vi "Client UI.vi"(8 "error in (no error)":errorcluster, 11 "Chat Client in":refnum<class "Chat Client.lvclass">) -> (0 "error out":errorcluster, 3 "Chat Client out":refnum<class "Chat Client.lvclass">)   [LabVIEW 2020, in "Chat Client.lvclass"]
uses:
  Chat Client.lvclass
  Chat Client.lvclass/Chat Client.ctl
  Stream-TCP/TCP Client/TCP Client.lvclass
panel:
  in  "Send":bool
  in  "Message":string
  out "Log":string
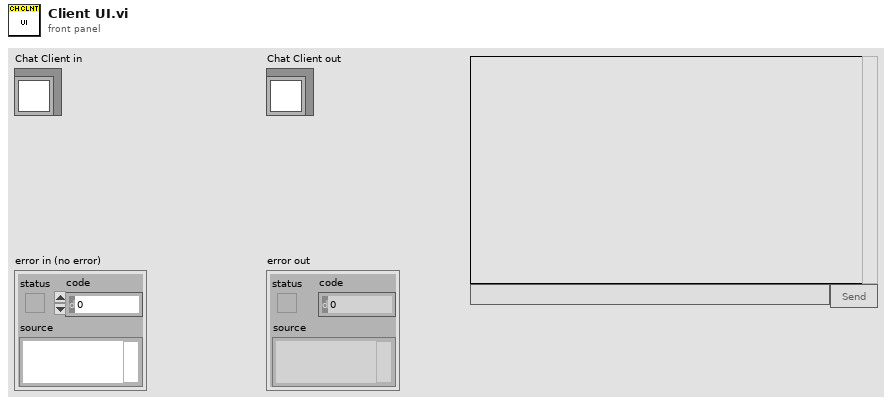
[diagram p1: front panel]
types:
  T1 = enum8{"Enabled", "Disabled", "Disabled and Grayed Out"}
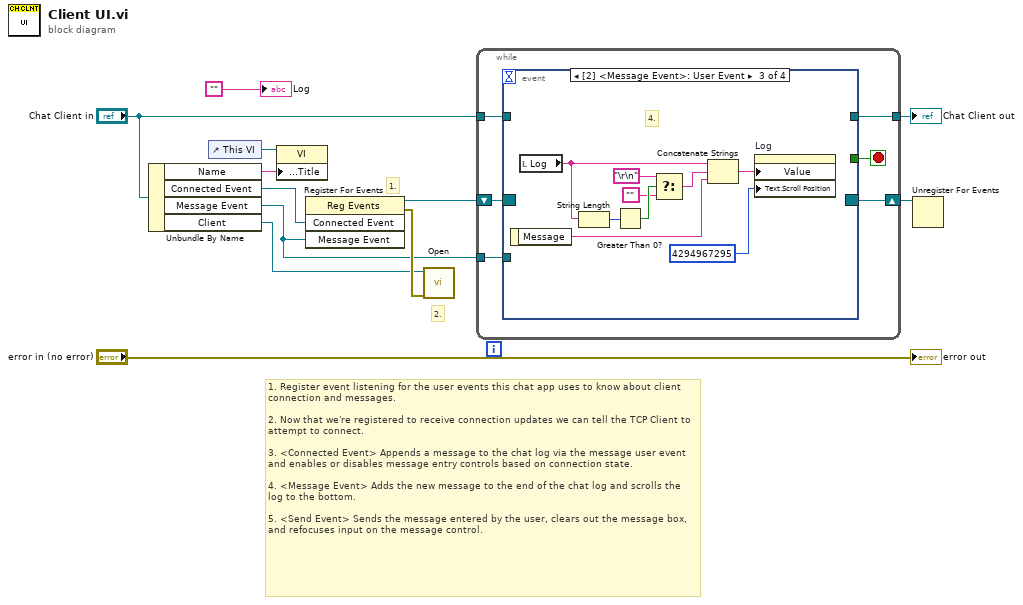
[diagram p0: block diagram]
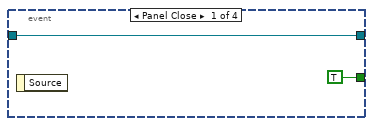
[diagram p2: hidden frame]
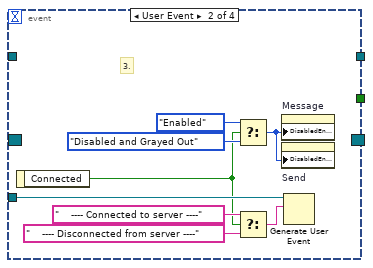
[diagram p3: hidden frame]
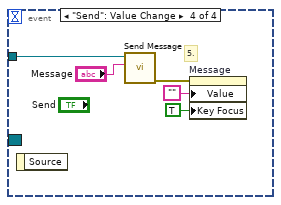
[diagram p4: hidden frame]
diagram:
  # "1. Register event listening for the user events this chat app uses to know about client connection and messages.\n\n2. Now that we're registered to receive connection updates we can tell the TCP Client to attempt to connect.\n\n3. <Connected Event> Appends a message to the chat log via the message user event and enables or disables message entry controls based on connection state.\n\n4. <Message Event> Adds the new message to the end of the chat log and scrolls the log to the bottom.\n\n5. <Send Event> Sends the message entered by the user, clears out the message box, and refocuses input on the message control."
  # "2."
  # "1."
  n1 = Unbundle By Name("Chat Client in") -> ("Name"=w9:string, "Connected Event"=w8:refnum<user-event>, "Message Event"=w5:refnum<user-event>, "Client"=w1:refnum<class "TCP Client.lvclass">)
  n2 = control-ref of="This VI"() -> (w10:refnum<vi>)
  n3 = property class="VI"(reference=w10, "Front Panel.Title"=w9) -> ()  [unwired: 1 in, 2 out]
  n4 = register-events(w8, w5) -> (reference out=w7:refnum<event-registration>, error out=w12:errorcluster)  [unwired: 2 in]
  n5 = call-dynamic "Open.vi"("error in (no error)"=w12, "TCP Client in"=w1) -> ()  [unwired: 8 in, 2 out]
  n6 = while {
    shift-right: [w16] -> w6
    shift-left: w7 -> [w18]
    tunnel: w5 -> [w15]
    tunnel: "Chat Client in" -> [w14]
    tunnel: [w13] -> w3
    stop <- w17 stop-if-true
    n7 = event shown="[2] <Message Event>: User Event" {
      selector: w18 -> [_ _ _ _]
      dyn-events: [_ _ _ _] -> w16
      timeout: _ -> [_ _ _ _]
      tunnel: [TRUE _ _ _] -> w17
      tunnel: w15 -> [_ w28 _ _]
      tunnel: w14 -> [w19 _ _ w42]
      tunnel: [w19 _ _ _] -> w13
      event Panel Close {
        n8 = event-data() -> ()  [unwired: 1 in, 1 out]
      }
      event User Event {
        # "3."
        n9 = event-data() -> ("Connected"=w22:bool)  [unwired: 1 in]
        n10 = Select(t=T1."Enabled" ("Disabled"), s=w22, f=T1."Disabled and Grayed Out" ("Disabled")) -> (s? t:f=w21:T1)
        n11 = Select(t="    ---- Connected to server ----", s=w22, f="    ---- Disconnected from server ----") -> (s? t:f=w25:string)
        n12 = property on="Message" class="Str"("DisabledEnum"=w21) -> ()  [unwired: 2 in, 2 out]
        n13 = property on="Send" class="Bool"("DisabledEnum"=w21) -> ()  [unwired: 2 in, 2 out]
        n14 = Generate User Event(user event=w28, event data cluster=w25) -> ()  [unwired: 2 in, 2 out]
      }
      event User Event {
        # "4."
        n15 = event-data() -> ("Message"=w31:string)  [unwired: 1 in]
        n16 = local read "Log"() -> (w37:string)
        n17 = String Length(string=w37) -> (length=w36:i32)
        n18 = Greater Than 0?(x=w36) -> (x > 0?=w35:bool)
        n19 = Select(t="\r\n", s=w35, f="") -> (s? t:f=w32:string)
        n20 = Concatenate Strings(w37, w32, w31) -> (w30:string)
        n21 = property on="Log" class="Str"("Value"=w30, "Text.Scroll Position"=u32 4294967295) -> ()  [unwired: 2 in, 2 out]
      }
      event "Send": Value Change {
        # "5."
        n22 = event-data() -> ()  [unwired: 1 in, 1 out]
        n23 = call "Send Message.vi"("Message"="Message", "Chat Client in"=w42) -> ("error out"=w40:errorcluster)  [unwired: 8 in, 1 out]
        n24 = property on="Message" class="Str"(error in=w40, "Value"="", "Key Focus"=TRUE) -> ()  [unwired: 1 in, 2 out]
      }
    }
  }
  "Chat Client out" <- w3
  n25 = Unregister For Events(event registration refnum=w6) -> ()  [unwired: 1 in, 1 out]
  "error out" <- "error in (no error)"
  "Log" <- ""
